vi "Demo.vi"() -> ()   [LabVIEW 2018, in "Config.lvlib"]
uses:
  Config.lvlib
  096bbc21-a282-466f-94f4-9dc436c1a68c.vi
  33a24eb8-ecb5-48b8-a0e8-18e05276a395.vi
  886381bb-8ffb-46a9-98ee-47564b5ad809.vi
  f56f3c72-021e-4d67-8059-f7a679179f11.vi
panel:
  out "Key2 Found?":bool
  out "Key2 Value":i32
  out "Remove Section?":bool
  out "Remove Key?":bool
  out "Section Found?":bool
  out "Keys":string[](array[string])
  out "Sections":string[](array[string])
  out "Key1 Found?":bool
  out "Key1 Value":string
  out "error out":errorcluster
  out "All Keys":T1(array[cluster])
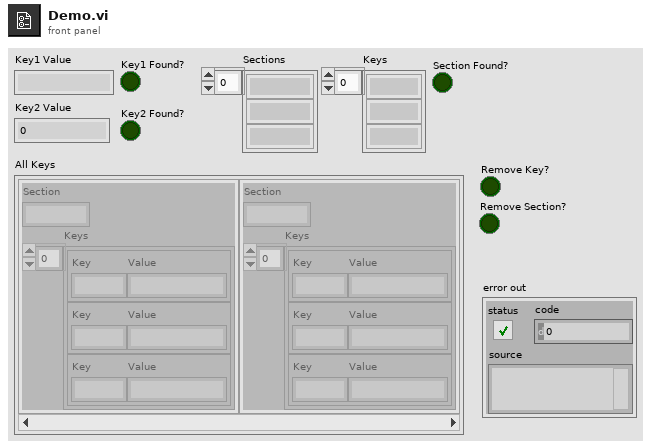
[diagram p1: front panel]
types:
  T1 = cluster{"Section":string, "Keys":cluster{"Key":string, "Value":string}[]}[]
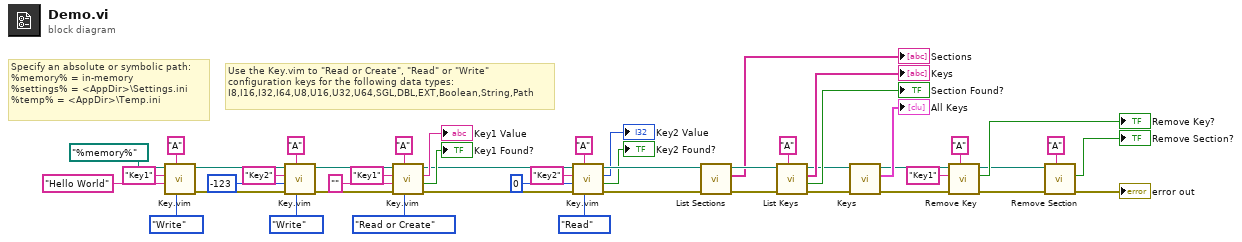
[diagram p0: block diagram]
diagram:
  # "Use the Key.vim to \"Read or Create\", \"Read\" or \"Write\"\nconfiguration keys for the following data types:\nI8,I16,I32,I64,U8,U16,U32,U64,SGL,DBL,EXT,Boolean,String,Path"
  # "Specify an absolute or symbolic path:\n%memory% = in-memory\n%settings% = <AppDir>\\Settings.ini\n%temp% = <AppDir>\\Temp.ini"
  n1 = call "Key.vim"("Operation (Read or Create)"=enum8{"Read or Create", "Read", "Write"}."Write", "Section"="A", "Value"="Hello World", "Key"="Key1", "Ini Path in"=path "%memory%") -> ("error out"=w46:errorcluster, "Ini Path out"=w43:path)  [unwired: 3 in, 2 out]
  n2 = call "Key.vim"("Operation (Read or Create)"=enum8{"Read or Create", "Read", "Write"}."Write", "Section"="A", "error in (no error)"=w46, "Value"=-123, "Key"="Key2", "Ini Path in"=w43) -> ("error out"=w33:errorcluster, "Ini Path out"=w1:path)  [unwired: 2 in, 2 out]
  n3 = call "Key.vim"("Operation (Read or Create)"=enum8{"Read or Create", "Read", "Write"}."Read or Create", "Section"="A", "error in (no error)"=w33, "Value"="", "Key"="Key1", "Ini Path in"=w1) -> ("error out"=w26:errorcluster, "Found?"=→"Key1 Found?":bool, "Value out"=→"Key1 Value":string, "Ini Path out"=w25:path)  [unwired: 2 in]
  n4 = call "Key.vim"("Operation (Read or Create)"=enum8{"Read or Create", "Read", "Write"}."Read", "Section"="A", "error in (no error)"=w26, "Value"=0, "Key"="Key2", "Ini Path in"=w25) -> ("error out"=w20:errorcluster, "Found?"=→"Key2 Found?":bool, "Value out"=→"Key2 Value":i32, "Ini Path out"=w21:path)  [unwired: 2 in]
  n5 = call "List Sections.vi"("error in (no error)"=w20, "Ini Path in"=w21) -> ("error out"=w23:errorcluster, "Sections"=→"Sections":string[], "Ini Path out"=w22:path)  [unwired: 7 in]
  n6 = call "List Keys.vi"("Section"="A", "error in (no error)"=w23, "Ini Path in"=w22) -> ("error out"=w15:errorcluster, "Section Found?"=→"Section Found?":bool, "Keys"=→"Keys":string[], "Ini Path out"=w14:path)  [unwired: 5 in]
  n7 = call "Keys.vi"("error in (no error)"=w15, "Ini Path in"=w14) -> ("error out"=w13:errorcluster, "Sections"=→"All Keys":T1, "Ini Path out"=w12:path)  [unwired: 7 in]
  n8 = call "Remove Key.vi"("Section"="A", "error in (no error)"=w13, "Key"="Key1", "Ini Path in"=w12) -> ("error out"=w9:errorcluster, "Key Found?"=→"Remove Key?":bool, "Ini Path out"=w2:path)  [unwired: 5 in]
  n9 = call "Remove Section.vi"("Section"="A", "error in (no error)"=w9, "Ini Path in"=w2) -> ("error out"=→"error out":errorcluster, "Section Found?"=→"Remove Section?":bool)  [unwired: 6 in, 1 out]
